vi "Combine PNGs two columns.vi"(8 "error in (no error)":errorcluster, 9 "Output File":path, 10 "Right Column":path[](array[path]), 11 "Left Column":path[](array[path])) -> (0 "error out":errorcluster)   [LabVIEW 2015, in "VIDiff_Screenshots.lvlib"]
uses:
  ImageMagic/Append Method.ctl
  VIDiff_Screenshots.lvlib
  ImageMagic/VIDiff_ImageMagic.lvlib
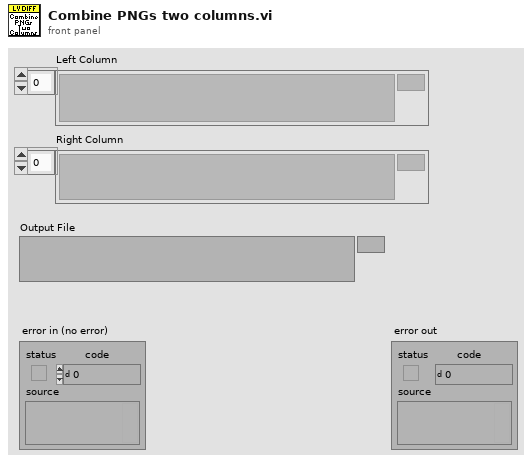
[diagram p1: front panel]
types:
  T1 = typedef "VIDiff_ImageMagic.lvlib/Append Method.ctl" = enum16{"Vertical", "Horizontal"}
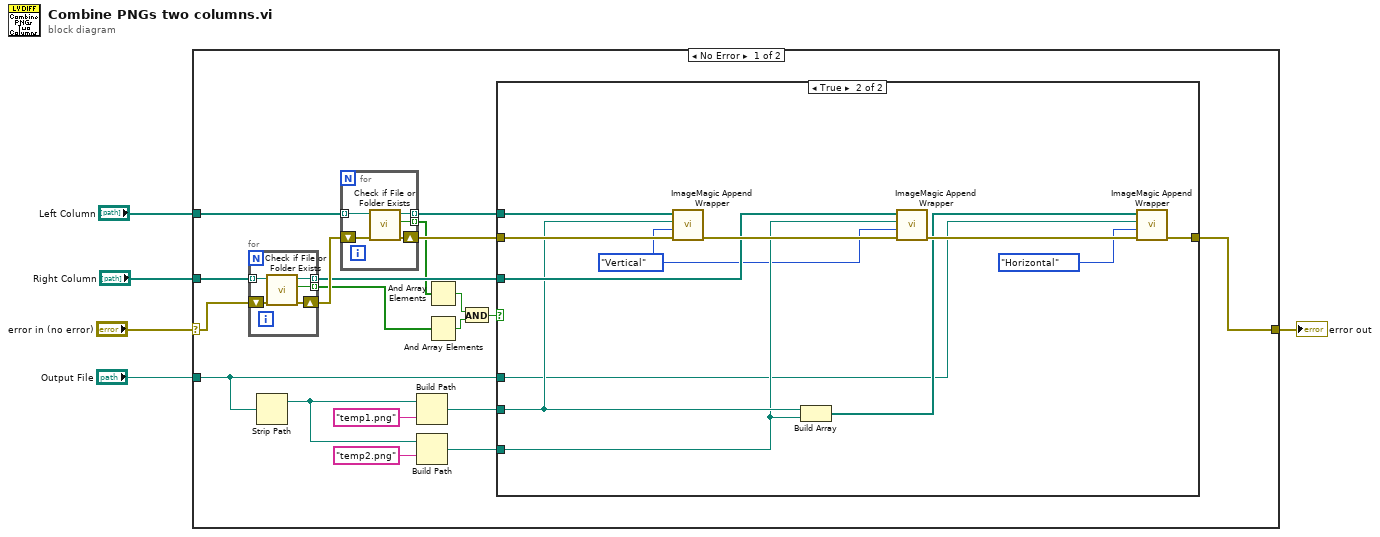
[diagram p0: block diagram]
diagram:
  n1 = case shown="No Error" "error in (no error)" {
    selector: "error in (no error)" -> [w21 w48]
    tunnel: [w24 w48] -> w4
    tunnel: "Left Column" -> [w17 _]
    tunnel: "Right Column" -> [w18 _]
    tunnel: "Output File" -> [w6 _]
    frame No Error {
      n2 = for {
        tunnel: [w32] -> w15 mode=indexing
        tunnel: [w31] -> w19 mode=indexing
        shift-right: [w33] -> w20
        shift-left: w21 -> [w34]
        tunnel: w18 -> [w30] mode=indexing
        n3 = call <vilib>:"Check if File or Folder Exists.vi"("error in (no error)"=w34, "path"=w30) -> ("error out"=w33:errorcluster, "file or folder exists?"=w32:bool, "dup path"=w31:path)  [unwired: 7 in]
      }
      n4 = Strip Path(path=w6) -> (stripped path=w11:path)  [unwired: 1 out]
      n5 = for {
        tunnel: [w29] -> w23 mode=indexing
        tunnel: w17 -> [w26] mode=indexing
        shift-right: [w28] -> w22
        shift-left: w20 -> [w27]
        tunnel: [w25] -> w16 mode=indexing
        n6 = call <vilib>:"Check if File or Folder Exists.vi"("error in (no error)"=w27, "path"=w26) -> ("error out"=w28:errorcluster, "file or folder exists?"=w25:bool, "dup path"=w29:path)  [unwired: 7 in]
      }
      n7 = Build Path(base path=w11, name or relative path="temp1.png") -> (appended path=w8:path)
      n8 = Build Path(base path=w11, name or relative path="temp2.png") -> (appended path=w7:path)
      n9 = And Array Elements(Boolean array=w16) -> (logical AND=w13:bool)
      n10 = And Array Elements(Boolean array=w15) -> (logical AND=w14:bool)
      n11 = And(x=w13, y=w14) -> (x .and. y?=w12:bool)
      n12 = case shown="True" w12 {
        tunnel: w23 -> [_ w46]
        tunnel: w19 -> [_ w44]
        tunnel: w22 -> [w35 w47]
        tunnel: [w35 w38] -> w24
        tunnel: w8 -> [_ w42]
        tunnel: w7 -> [_ w41]
        tunnel: w6 -> [_ w39]
        frame False {
        }
        frame True {
          w37 = Append_Method."Vertical" ("Append Method")
          n13 = call "ImageMagic Append Wrapper.vi"("error in (no error)"=w47, "Append Method"=w37, "Output File"=w42, "Input Files"=w46) -> ("error out"=w45:errorcluster)  [unwired: 7 in]
          n14 = Build Array(w42, w41) -> (w40:path[])
          n15 = call "ImageMagic Append Wrapper.vi"("error in (no error)"=w45, "Append Method"=w37, "Output File"=w41, "Input Files"=w44) -> ("error out"=w43:errorcluster)  [unwired: 7 in]
          n16 = call "ImageMagic Append Wrapper.vi"("error in (no error)"=w43, "Append Method"=Append_Method."Horizontal", "Output File"=w39, "Input Files"=w40) -> ("error out"=w38:errorcluster)  [unwired: 7 in]
        }
      }
    }
    frame Error {
    }
  }
  "error out" <- w4
